vi "FTW-WebService-AwaitAndFinalize.vi"(0 "FTW Web Request":refnum<class "FTW-WebService.lvclass">, 5 "Timeout":i32 format="%dmsec", 11 "error in":errorcluster) -> (15 "error out":errorcluster)   [LabVIEW 2013, in "FTW-WebService.lvclass"]
uses:
  FTW-WebService.lvclass
  FTW-HTTP-ResponseCode.ctl
  FTW-WebService.lvclass/FTW-WebService.ctl
  <vilib>/wsapi/Web Request.lvclass
panel:
  # "Inputs"
  # "Outputs"
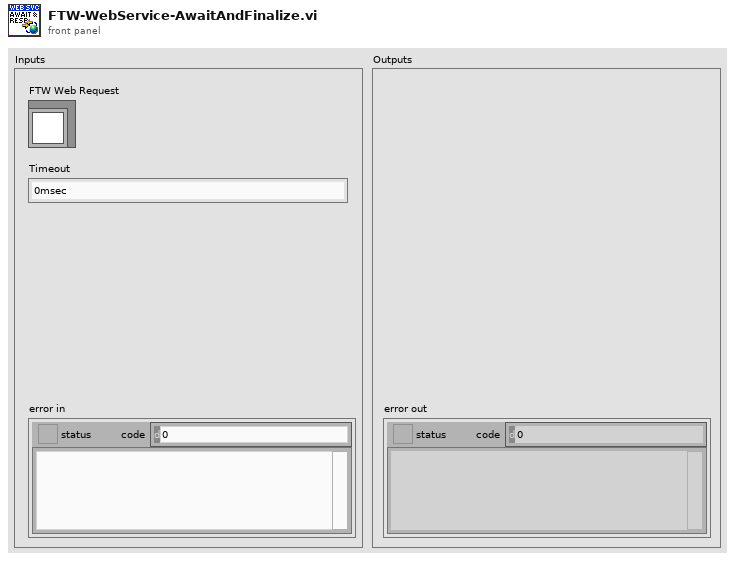
[diagram p1: front panel]
types:
  T1 = typedef "FTW-HTTP-ResponseCode.ctl" = i32
  T2 = typedef "FTW-WebService-Response.ctl" = cluster{"HTTP Response Code":T3, "Response Body":string}
  T3 = typedef "FTW-Web-HTTPResponseCode.ctl" = i32
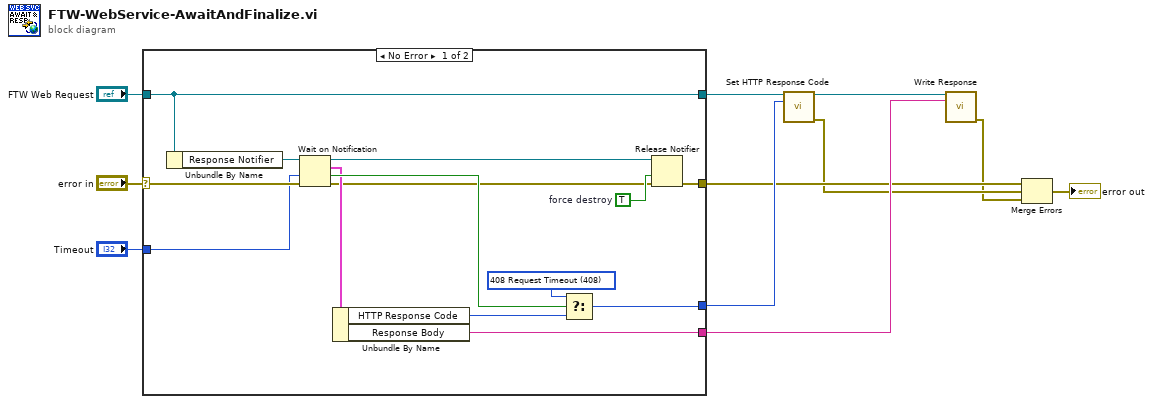
[diagram p0: block diagram]
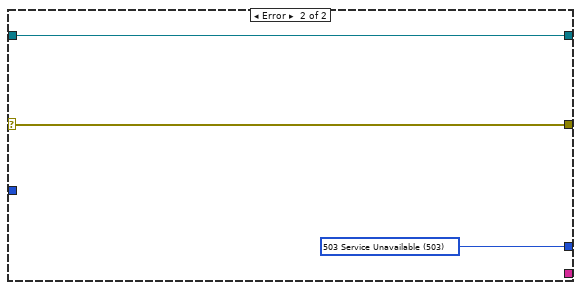
[diagram p2: hidden frame]
diagram:
  n1 = case shown="No Error" "error in" {
    selector: "error in" -> [w25 w27]
    tunnel: [w22 w28] -> w9
    tunnel: [w17 _] -> w8
    tunnel: [w12 w27] -> w7
    tunnel: [w21 w26] -> w4
    tunnel: "FTW Web Request" -> [w21 w26]
    tunnel: "Timeout" -> [w19 _]
    frame No Error {
      w14 = TRUE  # force destroy
      w23 = T1 408 items=["100 Continue"=100, "101 Switching Protocols"=101, "200 OK"=200, "201 Created"=201, "202 Accepted"=202, "203 Non-Authoritative Information"=203, "204 No Content"=204, "205 Reset Content"=205, "206 Partial Content"=206, "300 Multiple Choices"=300, "301 Moved Permanently"=301, "302 Found"=302, "303 See Other"=303, "304 Not Modified"=304, "305 Use Proxy"=305, "306 (Unused)"=306, "307 Temporary Redirect"=307, "400 Bad Request"=400, "401 Unauthorized"=401, "402 Payment Required"=402, "403 Forbidden"=403, "404 Not Found"=404, "405 Method Not Allowed"=405, "406 Not Acceptable"=406, "407 Proxy Authentication Required"=407, "408 Request Timeout"=408, "409 Conflict"=409, "410 Gone"=410, "411 Length Required"=411, "412 Precondition Failed"=412, "413 Request Entity Too Large"=413, "414 Request-URI Too Long"=414, "415 Unsupported Media Type"=415, "416 Requested Range Not Satisfiable"=416, "417 Expectation Failed"=417, "500 Internal Server Error"=500, "501 Not Implemented"=501, "502 Bad Gateway"=502, "503 Service Unavailable"=503, "504 Gateway Timeout"=504, "505 HTTP Version Not Supported"=505] ("HTTP Response Code")
      n2 = Unbundle By Name(w21) -> ("Response Notifier"=w20:refnum<notifier>)
      n3 = Wait on Notification(notifier=w20, timeout in ms (-1)=w19, error in (no error)=w25) -> (notifier out=w15:refnum<notifier>, notification=w18:T2, timed out?=w24:bool, error out=w13:errorcluster)  [unwired: 1 in]
      n4 = Unbundle By Name(w18) -> ("HTTP Response Code"=w16:T3, "Response Body"=w17:string)
      n5 = Select(t=w23, s=w24, f=w16) -> (s? t:f=w22:T3)
      n6 = Release Notifier(notifier=w15, force destroy? (F)=w14, error in (no error)=w13) -> (error out=w12:errorcluster)  [unwired: 2 out]
    }
    frame Error {
      w28 = T1 503 items=["100 Continue"=100, "101 Switching Protocols"=101, "200 OK"=200, "201 Created"=201, "202 Accepted"=202, "203 Non-Authoritative Information"=203, "204 No Content"=204, "205 Reset Content"=205, "206 Partial Content"=206, "300 Multiple Choices"=300, "301 Moved Permanently"=301, "302 Found"=302, "303 See Other"=303, "304 Not Modified"=304, "305 Use Proxy"=305, "306 (Unused)"=306, "307 Temporary Redirect"=307, "400 Bad Request"=400, "401 Unauthorized"=401, "402 Payment Required"=402, "403 Forbidden"=403, "404 Not Found"=404, "405 Method Not Allowed"=405, "406 Not Acceptable"=406, "407 Proxy Authentication Required"=407, "408 Request Timeout"=408, "409 Conflict"=409, "410 Gone"=410, "411 Length Required"=411, "412 Precondition Failed"=412, "413 Request Entity Too Large"=413, "414 Request-URI Too Long"=414, "415 Unsupported Media Type"=415, "416 Requested Range Not Satisfiable"=416, "417 Expectation Failed"=417, "500 Internal Server Error"=500, "501 Not Implemented"=501, "502 Bad Gateway"=502, "503 Service Unavailable"=503, "504 Gateway Timeout"=504, "505 HTTP Version Not Supported"=505] ("HTTP Response Code")
    }
  }
  n7 = call <vilib>:"Set HTTP Response Code.vi"("LabVIEW Web Service Request"=w4, "response code (200)"=w9) -> ("LabVIEW Web Service Request out"=w11:refnum<class "FTW-WebService.lvclass">, "error out"=w6:errorcluster)  [unwired: 12 in]
  n8 = call <vilib>:"Write Response.vi"("LabVIEW Web Service Request"=w11, "response string"=w8) -> ("error out"=w5:errorcluster)  [unwired: 12 in, 1 out]
  n9 = Merge Errors(w7, w6, w5) -> (→"error out":errorcluster)
